vi "Ex3Task2_Main.vi"() -> ()   [LabVIEW 2014, in "Ex3Task2_SA.lvrbt"]
uses:
  Ex3Task2_SA.lvrbt
  <vilib>/NXT/Block Support/NXT_InputPort.ctl
  <vilib>/NXT/Block Support/NXT_OutputPort.ctl
  <vilib>/NXT/Dual Mode Library/Sensors/EV3_Ultrasonic_CM.vi
  <vilib>/NXT/NXTIO Xnodes/NXTIONodeSubVIs/NXTMoveMotors.vi
  <vilib>/NXT/Subs/LVHSConnector.ctl
  <vilib>/NXT/NXTIO Xnodes/AddressXNode/NXTIOAddress.xnode
  <vilib>/NXT/NXTIO Xnodes/NXTIOXNode/NXTIO.xnode
  <vilib>/NXT/LegoClasses/BrickReference/BrickReference.lvclass
panel:
  in  "Stop Button":bool
  out "Distance From Wall":dbl
  out "Number of Loop Iterations":i32
  out "Final Iteration Value":i32
  out "Current Iteration":i32
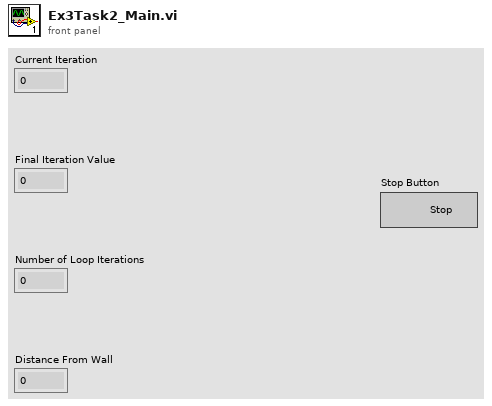
[diagram p1: front panel]
types:
  T1 = typedef "NXT_OutputPort.ctl" = u8
  T2 = typedef "NXT_InputPort.ctl" = u32
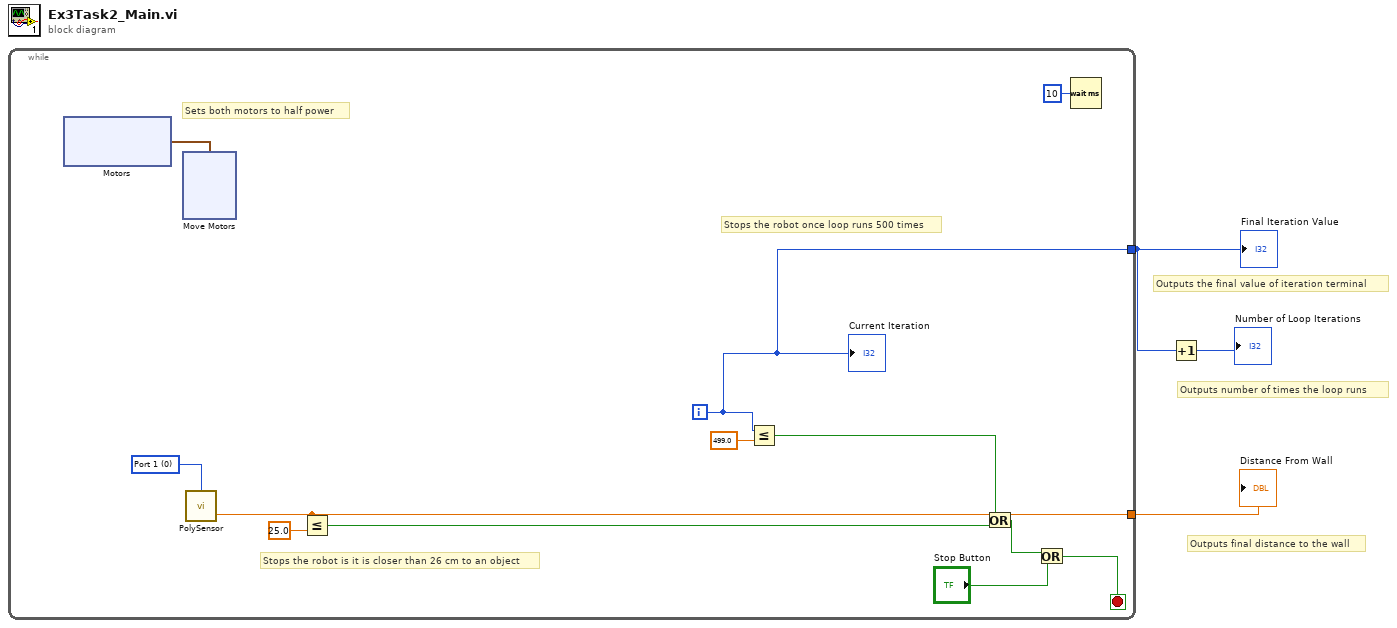
[diagram p0: block diagram]
diagram:
  # "Outputs the final value of iteration terminal"
  # "Outputs number of times the loop runs"
  # "Outputs final distance to the wall"
  n1 = while {
    tunnel: [w6] -> w2
    tunnel: [w5] -> w3
    i -> [w6]
    stop <- w12 stop-if-true
    w14 = T2 0 items=["Port 1", "Port 2", "Port 3", "Port 4"] ("Port (Port 1)")
    # "Stops the robot is it is closer than 26 cm to an object"
    # "Stops the robot once loop runs 500 times"
    # "Sets both motors to half power"
    n2 = xnode "Motors"() -> ("Motor"=w15:cluster{"Port":T1, "Port":T1})
    n3 = xnode "Move Motors"("Motors"=w15) -> ()  [unwired: 3 in, 1 out]
    n4 = call-poly <vilib>:"PolySensor.vi"("Port (Port 1)"=w14) -> ("Centimeters"=w5:sgl)  [unwired: 2 in, 1 out]
    n5 = Less Or Equal?(x=w5, y=sgl 25.0) -> (x <= y?=w9:bool)
    n6 = Less Or Equal?(x=w6, y=499.0) -> (x <= y?=w7:bool)
    n7 = Or(x=w7, y=w9) -> (x .or. y?=w11:bool)
    n8 = Or(x=w11, y="Stop Button") -> (x .or. y?=w12:bool)
    n9 = Wait (ms)(milliseconds to wait=u32 10) -> ()  [unwired: 1 out]
    "Current Iteration" <- w6
  }
  "Final Iteration Value" <- w2
  "Distance From Wall" <- w3
  n10 = Increment(x=w2) -> (x+1=→"Number of Loop Iterations":i32)
